vi "Update_TS_Parameter.vi"(8 "error in (no error)":errorcluster, 10 "TS Parameter":T2={"ProfitCenterCode"="5Y5676", "LineCode"="L07", "WorkOrderNumber"="66456", "Model"="29032639", "Model_with_Prefix"="0029032639", "VendorCode"="BD02", "SetParameterDateCode"="12Bj", "PokaYoke"=0, "Target"=200, "Live_DateCode"="12Bj", "CustomerPartNumber"="475465464", "Hose_Type"="FRONT", "sBarcode"=FALSE, "FCA"=3, "Ent_Stamp"=timestamp(0 s since 1904-01-01), "STS_CD"=0.0} {"FCA" format="%01d"; "Target" min=1 max=100000; "PokaYoke" min=0 max=1}, 11 "Refnum in":T1) -> (0 "error out":errorcluster, 2 "INSERT Script":string, 3 "Refnum Out":T1)   [LabVIEW 2020]
uses:
  Controls/TS_Parameter_V2.ctl
  <vilib>/addons/database/Connection.llb/Conn ObjectReference.ctl
  <vilib>/addons/database/Connection.llb/Conn Execute.vi
  <vilib>/addons/database/Recordset.llb/Rec Destroy - Connection.vi
  <vilib>/addons/database/NI_Database_API.lvlib
panel:
  out "error out 2":errorcluster
  out "trimmed string":string
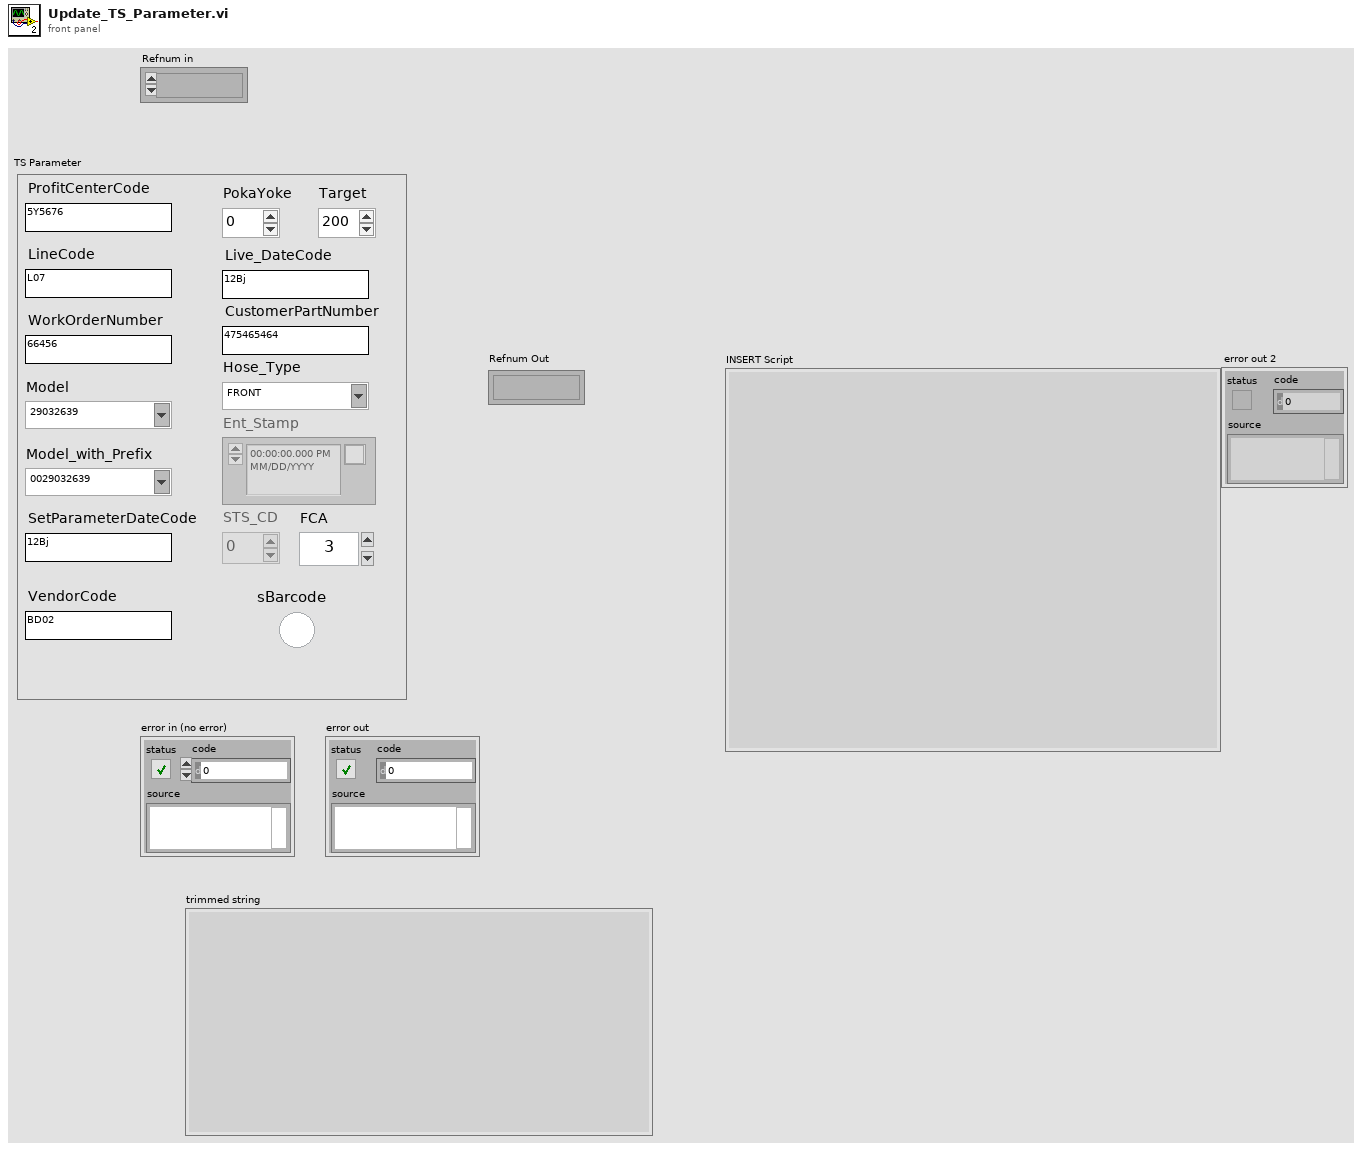
[diagram p1: front panel]
types:
  T1 = typedef "NI_Database_API.lvlib/Conn ObjectReference.ctl" = refnum<k1>
  T2 = typedef "TS_Parameter_V2.ctl" = cluster{"ProfitCenterCode":string, "LineCode":string, "WorkOrderNumber":string, "Model":string, "Model_with_Prefix":string, "VendorCode":string, "SetParameterDateCode":string, "PokaYoke":i32, "Target":i32, "Live_DateCode":string, "CustomerPartNumber":string, "Hose_Type":string, "sBarcode":bool, "FCA":i32, "Ent_Stamp":timestamp, "STS_CD":dbl}
  T3 = typedef "NI_Database_API.lvlib/Rec ObjectReference.ctl" = refnum<k1>
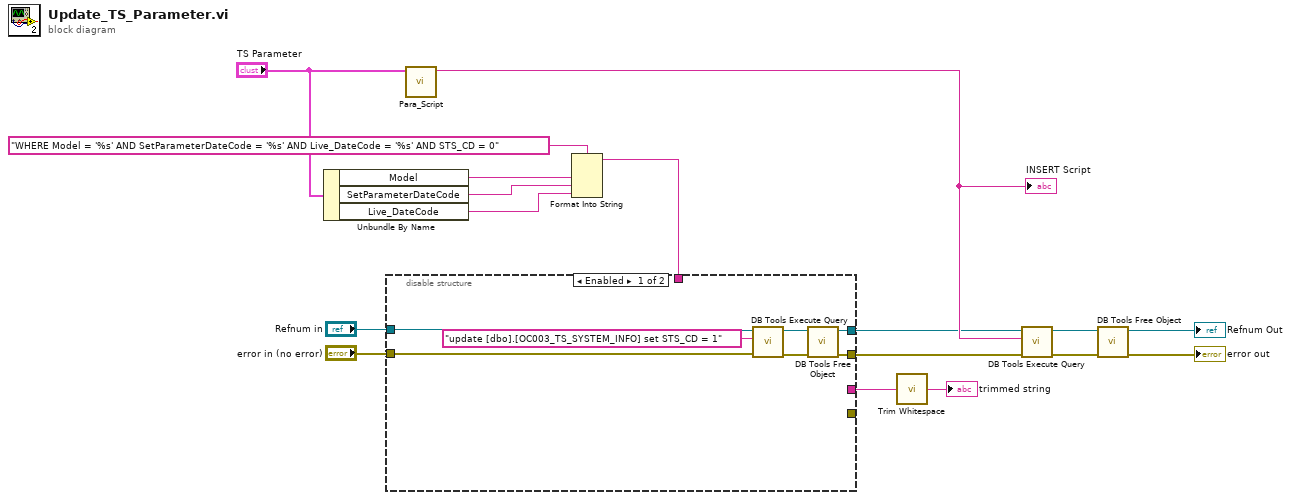
[diagram p0: block diagram]
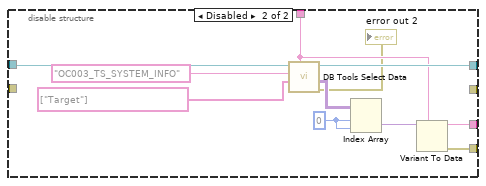
[diagram p2: hidden frame]
diagram:
  n1 = Unbundle By Name("TS Parameter") -> ("Model"=w7:string, "SetParameterDateCode"=w6:string, "Live_DateCode"=w5:string)
  n2 = call "Para_Script.vi"("TS Parameter"="TS Parameter") -> ("iNSERT Script"=w17:string)  [unwired: 9 in, 1 out]
  "INSERT Script" <- w17
  n3 = Format Into String(format string="WHERE Model = '%s' AND SetParameterDateCode = '%s' AND Live_DateCode = '%s' AND STS_CD = 0" ("ProfitCenterCode"), w7, w6, w5) -> (resulting string=w4:string)  [unwired: 2 in, 1 out]
  n4 = disable-structure shown="Enabled" {
    disable-tunnel: [w24 _] -> w16
    disable-tunnel: [w23 w34] -> w15
    disable-tunnel: "error in (no error)" -> [w19 _]
    disable-tunnel: "Refnum in" -> [w18 w35]
    disable-tunnel: w4 -> [_ w28]
    disable-tunnel: [_ w27] -> w3
    disable-tunnel: [_ w26] -> _
    frame Enabled {
      n5 = call-poly <vilib>:"DB Tools Execute Query.vi"("error in (no error)"=w19, "SQL query"="update [dbo].[OC003_TS_SYSTEM_INFO] set STS_CD = 1", "connection reference"=w18) -> ("error out"=w22:errorcluster, "recordset reference"=w21:T3)  [unwired: 5 in]
      n6 = call-poly <vilib>:"DB Tools Free Object.vi"("error in (no error)"=w22, "recordset reference"=w21) -> ("error out"=w24:errorcluster, "connection reference"=w23:T1)  [unwired: 8 in]
    }
    frame Disabled {
      w30 = 0 ("index (row)")
      n7 = call <vilib>:"DB Tools Select Data.vi"("condition"=w28, "columns"=string[] ["Target"], "table"="OC003_TS_SYSTEM_INFO", "connection reference"=w35) -> ("error out"=→"error out 2":errorcluster, "data"=w31:variant[][], "connection reference out"=w34:T1)  [unwired: 2 in]
      n8 = Index Array(array=w31, index (row)=w30, index (col)=w30) -> (element=w29:variant)
      n9 = Variant To Data(type=w28, Variant=w29) -> (data=w27:string, error out=w26:errorcluster)  [unwired: 1 in]
    }
  }
  n10 = call <vilib>:"Trim Whitespace.vi"("string"=w3) -> ("trimmed string"=→"trimmed string":string)  [unwired: 1 in]
  n11 = call-poly <vilib>:"DB Tools Execute Query.vi"("error in (no error)"=w16, "SQL query"=w17, "connection reference"=w15) -> ("error out"=w12:errorcluster, "recordset reference"=w13:T3)  [unwired: 5 in]
  n12 = call-poly <vilib>:"DB Tools Free Object.vi"("error in (no error)"=w12, "recordset reference"=w13) -> ("error out"=→"error out":errorcluster, "connection reference"=→"Refnum Out":T1)  [unwired: 8 in]
